vi "ServerGUI.vi"() -> ()   [LabVIEW 2009]
panel:
  in  "QUIT button":bool
  in  "Tab Control":T1(tab)
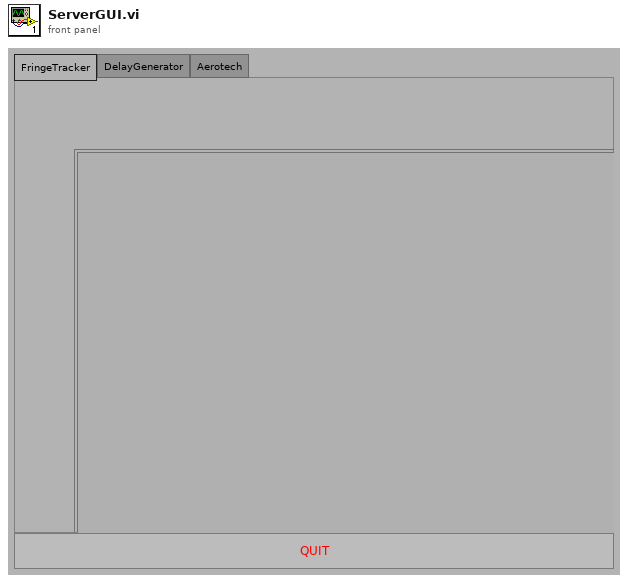
[diagram p1: front panel]
types:
  T1 = enum32{"Page 1", "Page 2", "Page 3", "Page 4", "Page 5", "Page 6", "Page 7"}
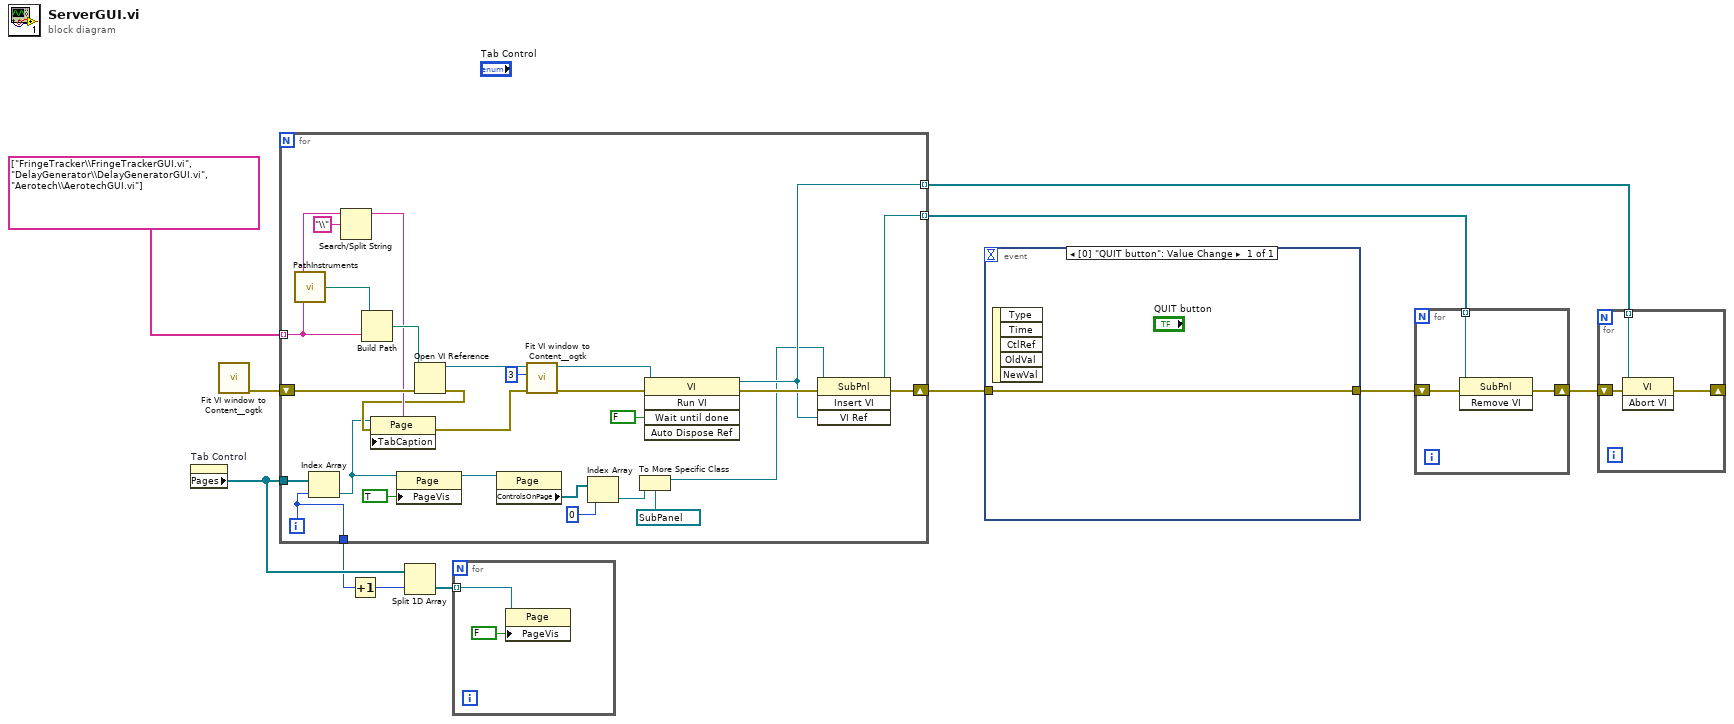
[diagram p0: block diagram]
diagram:
  n1 = property on="Tab Control" class="TabCtl (strict)"() -> ("Pages"=w4:refnum<vi>[])  [unwired: 2 in, 2 out]
  n2 = call <userlib>:"Fit VI window to Content__ogtk.vi"() -> ("error out"=w8:errorcluster)  [unwired: 6 in, 1 out]
  n3 = for {
    tunnel: [w34] -> w6 mode=indexing
    tunnel: [w33] -> w5 mode=indexing
    shift-right: [w35] -> w11
    shift-left: w8 -> [w27]
    tunnel: string[] ["FringeTracker\\FringeTrackerGUI.vi", "DelayGenerator\\DelayGeneratorGUI.vi", "Aerotech\\AerotechGUI.vi"] -> [w20] mode=indexing
    tunnel: w4 -> [w26]
    tunnel: [w15] -> w1
    i -> [w15]
    n4 = call "PathInstruments.vi"() -> ("Instruments Path"=w38:path)
    n5 = Index Array(array=w26, index=w15) -> (element=w12:refnum<vi>)
    n6 = Search/Split String(string=w20, search string/char (-)="\\") -> (substring before match=w18:string)  [unwired: 1 in, 2 out]
    n7 = Build Path(base path=w38, name or relative path=w20) -> (appended path=w37:path)
    n8 = property class="Page"(reference=w12, "PageVis"=TRUE ("Page Visible")) -> (reference out=w13:refnum<vi>)  [unwired: 1 in, 1 out]
    n9 = Open VI Reference(vi path=w37, error in (no error)=w27) -> (vi reference=w31:refnum<vi>, error out=w16:errorcluster)  [unwired: 4 in]
    n10 = property class="Page"(reference=w12, error in=w16, "TabCaption"=w18) -> (error out=w17:errorcluster)  [unwired: 1 out]
    n11 = property class="Page"(reference=w13) -> ("ControlsOnPage"=w25:refnum<vi>[])  [unwired: 1 in, 2 out]
    n12 = call <userlib>:"Fit VI window to Content__ogtk.vi"("error in (no error)"=w17, "border spacing (2 px)"=3, "VI Ref (calling VI)"=w31) -> ("error out"=w29:errorcluster, "dup VI Ref"=w30:refnum<vi>)  [unwired: 3 in]
    n13 = Index Array(array=w25, index=0) -> (element=w23:refnum<vi>)
    n14 = To More Specific Class(target class=refnum<vi> refnum ("Sub Panel Page1"), reference=w23) -> (specific class reference=w21:refnum<vi>)  [unwired: 1 in, 1 out]
    n15 = invoke class="VI" method="Run VI"(reference=w30, error in=w29, "Wait until done"=FALSE ("Wait Until Done")) -> (reference out=w33:refnum<vi>, error out=w36:errorcluster)  [unwired: 2 in, 3 out]
    n16 = invoke class="SubPnl" method="Insert VI"(reference=w21, error in=w36, "VI Ref"=w33) -> (reference out=w34:refnum<vi>, error out=w35:errorcluster)  [unwired: 1 in, 2 out]
  }
  n17 = Increment(x=w1) -> (x+1=w2:i32)
  n18 = Split 1D Array(array=w4, index=w2) -> (second subarray=w3:refnum<vi>[])  [unwired: 1 out]
  n19 = for {
    tunnel: w3 -> [w40] mode=indexing
    n20 = property class="Page"(reference=w40, "PageVis"=FALSE ("Page Visible")) -> ()  [unwired: 1 in, 2 out]
  }
  n21 = event shown="[0] \"QUIT button\": Value Change" {
    selector: _ -> [_]
    dyn-events: _ -> [_]
    timeout: _ -> [_]
    tunnel: w11 -> [w41]
    tunnel: [w41] -> w10
    event [0] "QUIT button": Value Change {
      n22 = event-data() -> ()  [unwired: 1 in, 5 out]
    }
  }
  n23 = for {
    shift-right: [w43] -> w9
    shift-left: w10 -> [w44]
    tunnel: w6 -> [w42] mode=indexing
    n24 = invoke class="SubPnl" method="Remove VI"(reference=w42, error in=w44) -> (error out=w43:errorcluster)  [unwired: 1 in, 2 out]
  }
  n25 = for {
    shift-right: [w46] -> _
    shift-left: w9 -> [w47]
    tunnel: w5 -> [w45] mode=indexing
    n26 = invoke class="VI" method="Abort VI"(reference=w45, error in=w47) -> (error out=w46:errorcluster)  [unwired: 1 in, 2 out]
  }
